vi "SwissSPAD Live_Launch FPGA Data Decoding Task.vi"(8 "error in (no error)":errorcluster, 9 "SwissSPAD Live Internal Variables":T1={"okCFrontPanelDevices Refnum"=refnum, "Bottom Device Refnum"=refnum, "Display Image"=refnum, "# Live Images"=0, "relative s"=0.0, "# Image Sets"=0, "Message"="", "Current Image Set"=0, "# Datasets in Series"=0, "Current Dataset"=0, "Live Mode"=FALSE, "Recording Mode"=FALSE, "Record Button"=refnum, "\nLive Button"=refnum, "SwissSPAD Live Gate Image Data Q Name"="", "Discard First Image"=FALSE, "Image Information"={"Save ROI Only"=FALSE, "Left"=0, "Top"=0, "Right"=0, "Bottom"=0, "Use Current ROI"=FALSE}, "Image Binning Options"={"Use Image Binning"=FALSE, "X Bin"=0, "Y Bin"=0}, "Bottom FPGA Serial Number"="", "Detector PCB Version"=enum."unknown", "# Acquisitions"=1, "10 bits"=FALSE, "Top FPGA Serial Number"="", "Top Device Refnum"=refnum, "okCFrontPanel Refnum"=refnum} {"# Acquisitions" min=1; "Image Binning Options"."Y Bin" min=1; "Image Binning Options"."X Bin" min=1}, 10 "Buffer Size (# 8-bit images)":i32) -> (0 "error out":errorcluster)   [LabVIEW 2021]
uses:
  SwissSPAD Live_Internal Variables.ctl
  D:/UCLA Thinkpad Google Drive/LabVIEW 2021 SP1/builds/SwissSPAD Live Distribution/Opal Kelly/C# Wrapper/v5.0.2/libFrontPanel-csharp.dll
  Opal Kelly/C# Wrapper/v5.0.2/libFrontPanel-csharp.dll
  <vilib>/vision/Image Controls.llb/IMAQ Image.ctl
  SwissSPAD Live_Image ROI Information.ctl
  Phasor/Image Binning Options.ctl
  SwissSPAD Live_SSx PCB Version.ctl
panel:
  out "created new Gate Image Data Q?":bool
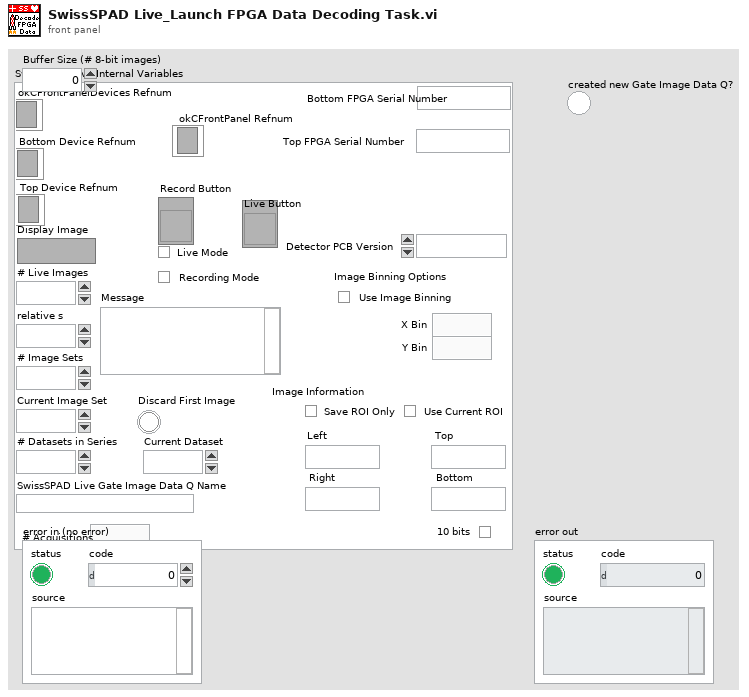
[diagram p1: front panel]
types:
  T1 = typedef "SwissSPAD Live_Internal Variables.ctl" = cluster{"okCFrontPanelDevices Refnum":refnum<k24>, "Bottom Device Refnum":refnum<k24>, "Display Image":T2, "# Live Images":i32, "relative s":dbl, "# Image Sets":i32, "Message":string, "Current Image Set":i32, "# Datasets in Series":i32, "Current Dataset":i32, "Live Mode":bool, "Recording Mode":bool, "Record Button":refnum<vi>, "\nLive Button":refnum<vi>, "SwissSPAD Live Gate Image Data Q Name":string, "Discard First Image":bool, "Image Information":T3, "Image Binning Options":T4, "Bottom FPGA Serial Number":string, "Detector PCB Version":T5, "# Acquisitions":u32, "10 bits":bool, "Top FPGA Serial Number":string, "Top Device Refnum":refnum<k24>, "okCFrontPanel Refnum":refnum<k24>}
  T2 = typedef "IMAQ Image.ctl" = refnum<image>
  T3 = typedef "SwissSPAD Live_Image ROI Information.ctl" = cluster{"Save ROI Only":bool, "Left":u16, "Top":u16, "Right":u16, "Bottom":u16, "Use Current ROI":bool}
  T4 = typedef "Image Binning Options.ctl" = cluster{"Use Image Binning":bool, "X Bin":i32, "Y Bin":i32}
  T5 = typedef "SwissSPAD Live_SSx PCB Version.ctl" = enum16{"unknown", "SS2 PCB1", "SS2 PCB2", "SS3 PCB1"}
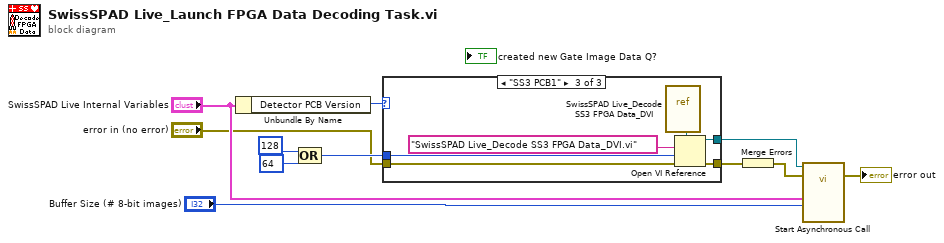
[diagram p0: block diagram]
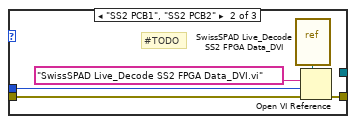
[diagram p3: hidden frame]
diagram:
  n1 = Unbundle By Name("SwissSPAD Live Internal Variables") -> ("Detector PCB Version"=w11:T5)
  n2 = Compound Arithmetic op=OR(128 ("options"), 64 ("options")) -> (w5:i32)
  n3 = case shown="\"SS3 PCB1\"" w11 {
    tunnel: w5 -> [_ w16 w22]
    tunnel: [_ _ w21] -> w6
    tunnel: [w12 w14 w20] -> w7
    tunnel: "error in (no error)" -> [w12 w13 w19]
    frame "unknown", Default {
    }
    frame "SS2 PCB1", "SS2 PCB2" {
      # "#TODO"
      n4 = vi-ref "SwissSPAD Live_Decode SS2 FPGA Data_DVI.vi"() -> (w15:refnum<vi>)
      n5 = Open VI Reference(type specifier VI Refnum (for type only)=w15, vi path="SwissSPAD Live_Decode SS2 FPGA Data_DVI.vi" ("Notebook Message"), options=w16, error in (no error)=w13) -> (error out=w14:errorcluster)  [unwired: 2 in, 1 out]
    }
    frame "SS3 PCB1" {
      n6 = vi-ref "SwissSPAD Live_Decode SS3 FPGA Data_DVI.vi"() -> (w18:refnum<vi>)
      n7 = Open VI Reference(type specifier VI Refnum (for type only)=w18, vi path="SwissSPAD Live_Decode SS3 FPGA Data_DVI.vi" ("Notebook Message"), options=w22, error in (no error)=w19) -> (vi reference=w21:refnum<vi>, error out=w20:errorcluster)  [unwired: 2 in]
    }
  }
  n8 = Merge Errors(w7) -> (w2:errorcluster)
  n9 = call-by-ref "Start Asynchronous Call"(reference=w6, error in=w2, "Buffer Size (# 8-bit Images)"="Buffer Size (# 8-bit images)", "SwissSPAD Live Internal Variables"="SwissSPAD Live Internal Variables") -> (error out=→"error out":errorcluster)  [unwired: 10 in, 1 out]
